vi "Check for Intersection.vi"(9 "Limits in":cluster{"Min":i64, "Max":i64}, 10 "Hailstone 2":refnum<class "Trace.lvclass">, 11 "Trace In":refnum<class "Trace.lvclass">) -> (3 "Boolean":bool)   [LabVIEW 2021, in "Trace.lvclass"]
uses:
  Trace/Trace.lvclass
  Trace/Trace.lvclass/Trace.ctl
  High Res Arithmetic/Rational Number.lvclass
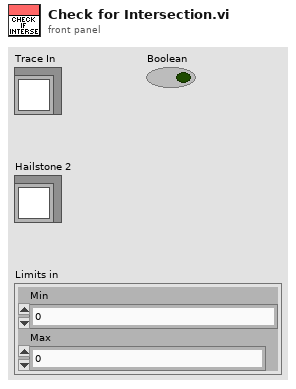
[diagram p1: front panel]
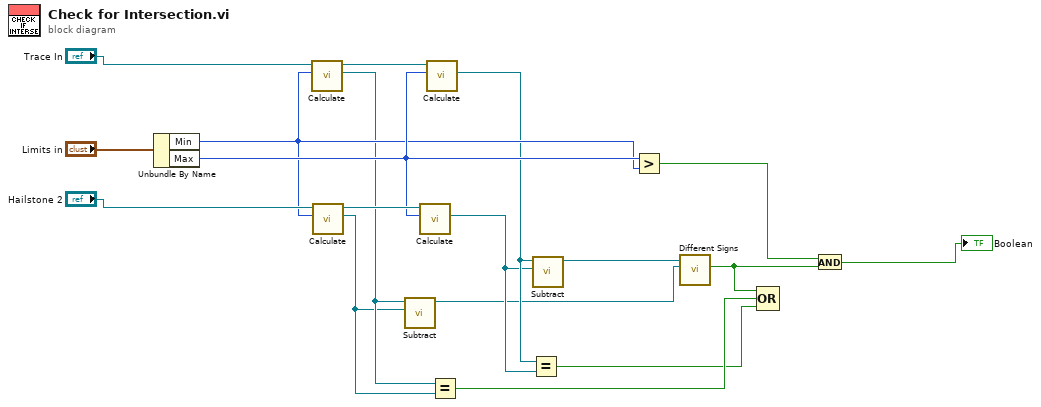
[diagram p0: block diagram]
diagram:
  n1 = Unbundle By Name("Limits in") -> ("Min"=w11:i64, "Max"=w12:i64)
  n2 = call "Calculate.vi"("X"=w11, "Trace in"="Trace In") -> ("Y"=w8:refnum<class "Rational Number.lvclass">, "Trace out"=w14:refnum<class "Trace.lvclass">)  [unwired: 7 in, 1 out]
  n3 = call "Calculate.vi"("X"=w11, "Trace in"="Hailstone 2") -> ("Y"=w7:refnum<class "Rational Number.lvclass">, "Trace out"=w15:refnum<class "Trace.lvclass">)  [unwired: 7 in, 1 out]
  n4 = call "Subtract.vi"("High Res Arithmetic 2"=w7, "High Res Arithmetic 1"=w8) -> ("High Res Arithmetic sum"=w2:refnum<class "Rational Number.lvclass">)  [unwired: 8 in, 1 out]
  n5 = call "Calculate.vi"("X"=w12, "Trace in"=w15) -> ("Y"=w4:refnum<class "Rational Number.lvclass">)  [unwired: 7 in, 2 out]
  n6 = call "Calculate.vi"("X"=w12, "Trace in"=w14) -> ("Y"=w5:refnum<class "Rational Number.lvclass">)  [unwired: 7 in, 2 out]
  n7 = Equal?(x=w8, y=w7) -> (x = y?=w6:bool)
  n8 = Equal?(x=w5, y=w4) -> (x = y?=w3:bool)
  n9 = call "Subtract.vi"("High Res Arithmetic 2"=w4, "High Res Arithmetic 1"=w5) -> ("High Res Arithmetic sum"=w9:refnum<class "Rational Number.lvclass">)  [unwired: 8 in, 1 out]
  n10 = Greater?(x=w12, y=w11) -> (0:w10:bool)
  n11 = call "Different Signs.vi"("High Res Arithmetic In 2"=w2, "High Res Arithmetic In"=w9) -> ("Different signs?"=w1:bool)  [unwired: 8 in, 1 out]
  n12 = Compound Arithmetic op=OR(w1, w6, w3) -> ()  [unwired: 1 out]
  n13 = And(x=w10, y=w1) -> (x .and. y?=→"Boolean":bool)
